vi "projet_modulation.vi"() -> ()   [LabVIEW 2026]
panel:
  out "Array":i32[](array[numeric])
  in  "modulation":enum16{"ASK", "PSK", "FSK"}(ring)
  in  "m":dbl
  in  "binary input":string
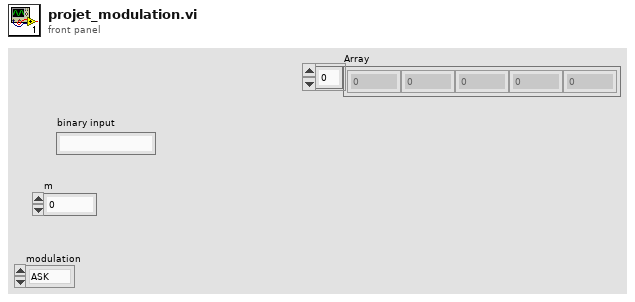
[diagram p1: front panel]
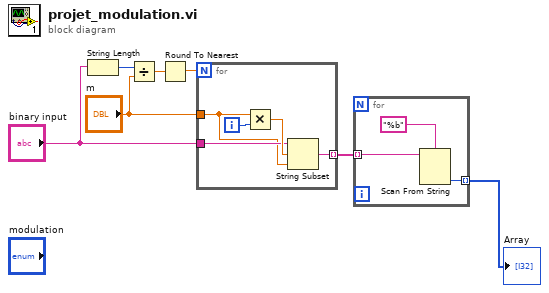
[diagram p0: block diagram]
diagram:
  n1 = String Length(string="binary input") -> (length=w7:i32)
  n2 = Divide(x=w7, y="m") -> (x/y=w6:dbl)
  n3 = Round To Nearest(number=w6) -> (nearest integer value=w5:dbl)
  n4 = for {
    N: w5 -> [_]
    tunnel: "m" -> [w9]
    tunnel: "binary input" -> [w10]
    tunnel: [w8] -> w2 mode=indexing
    i -> [w11]
    n5 = Multiply(x=w9, y=w11) -> (x*y=w12:dbl)
    n6 = String Subset(string=w10, offset (0)=w12, length (rest)=w9) -> (substring=w8:string)
  }
  n7 = for {
    tunnel: w2 -> [w14] mode=indexing
    tunnel: [w13] -> w1 mode=indexing
    n8 = Scan From String(format string="%b", input string=w14) -> (output 1=w13:i32)  [unwired: 3 in, 3 out]
  }
  "Array" <- w1
